vi "Main Screen_Hourly Cnt.vi"(9 "Current Date":string, 11 "connection reference 2":T1) -> (2 "Station Wise Max":i32[][](array[numeric]))   [LabVIEW 2017]
uses:
  <vilib>/addons/database/Connection.llb/Conn ObjectReference.ctl
  <vilib>/addons/database/Connection.llb/Conn Execute.vi
  <vilib>/addons/database/Recordset.llb/Rec Fetch Recordset Data (R).vi
  <vilib>/addons/database/Recordset.llb/Rec Destroy - Connection.vi
  <vilib>/addons/database/NI_Database_API.lvlib
panel:
  out "All Max":i32[](array[numeric])
  out "Table":string[][][](array[string])
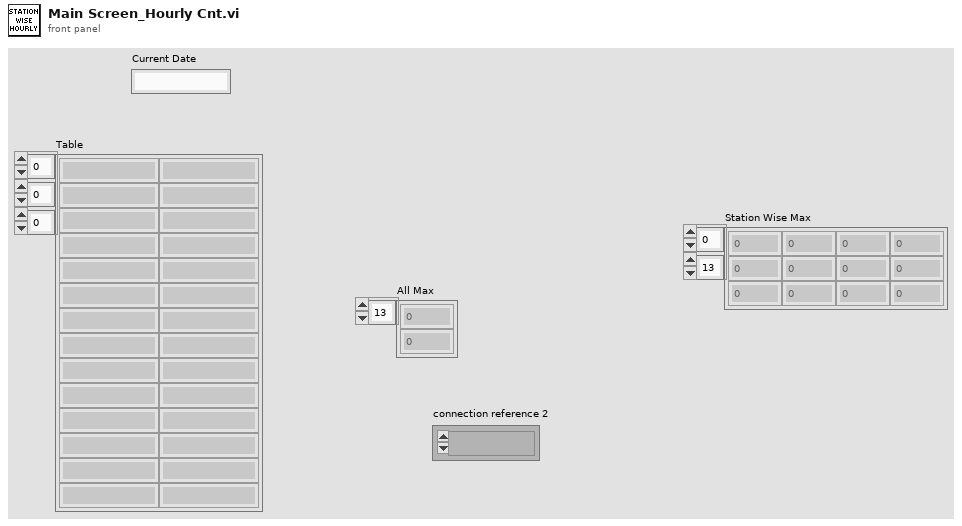
[diagram p1: front panel]
types:
  T1 = typedef "NI_Database_API.lvlib/Conn ObjectReference.ctl" = refnum<k1>
  T2 = typedef "NI_Database_API.lvlib/Rec ObjectReference.ctl" = refnum<k1>
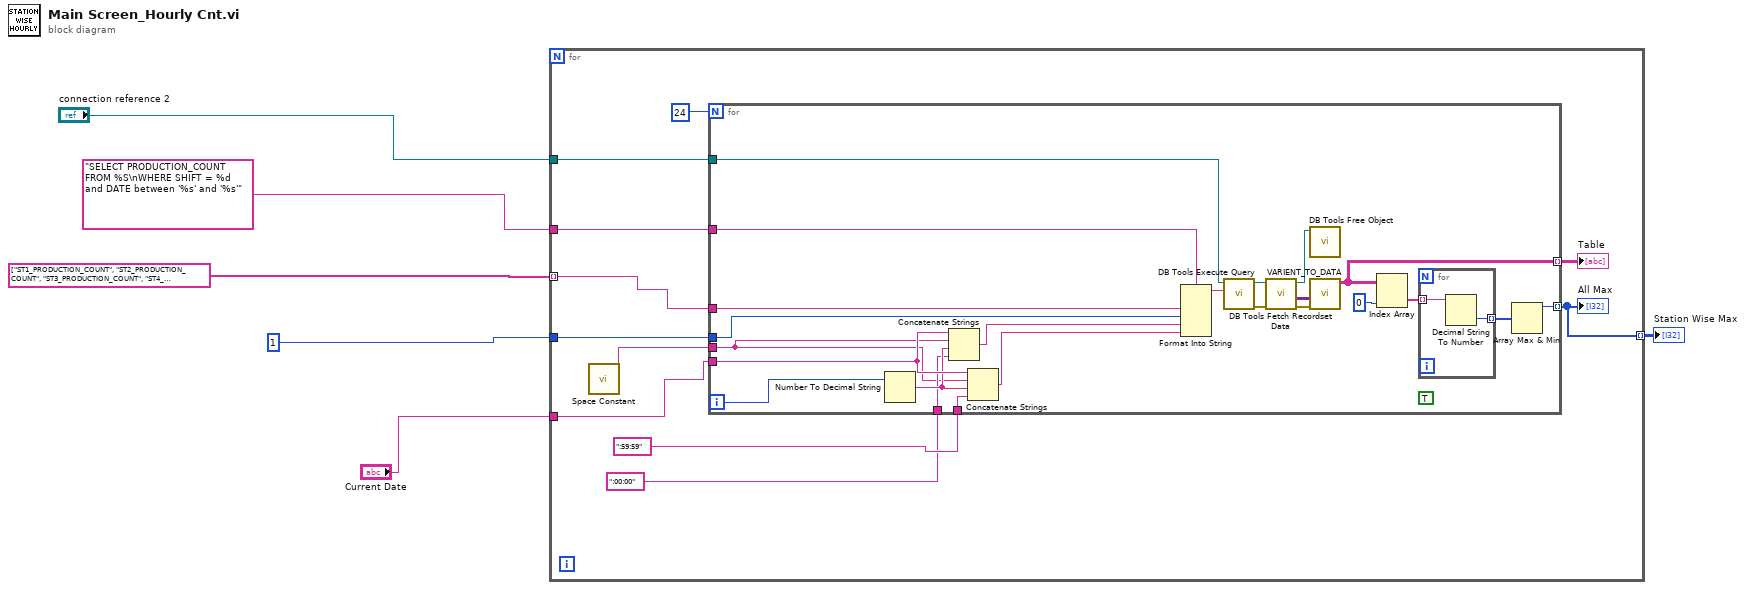
[diagram p0: block diagram]
diagram:
  n1 = for {
    tunnel: "SELECT PRODUCTION_COUNT FROM %S\nWHERE SHIFT = %d and DATE between '%s' and '%s'" ("SQL query") -> [w17]
    tunnel: 1 -> [w16]
    tunnel: "connection reference 2" -> [w15]
    tunnel: string[] ["ST1_PRODUCTION_COUNT", "ST2_PRODUCTION_COUNT", "ST3_PRODUCTION_COUNT", "ST4_PRODUCTION_COUNT", "ST5_PRODUCTION_COUNT", "ST6_PRODUCTION_COUNT"] -> [w10] mode=indexing
    tunnel: [w9] -> w2 mode=indexing
    tunnel: "Current Date" -> [w8]
    n2 = call <vilib>:"Space Constant.vi"() -> ("String"=w7:string)
    n3 = for {
      N: 24 -> [_]
      tunnel: w15 -> [w40]
      tunnel: w17 -> [w36]
      tunnel: w10 -> [w32]
      tunnel: w16 -> [w31]
      tunnel: w8 -> [w23]
      tunnel: [w29] -> w13 mode=indexing
      tunnel: [w30] -> w9 mode=indexing
      tunnel: ":59:59" -> [w24]
      tunnel: ":00:00" -> [w21]
      tunnel: w7 -> [w18]
      i -> [w19]
      (unwired) TRUE ("Check Hourly")
      n4 = Number To Decimal String(number=w19) -> (decimal integer string=w22:string)  [unwired: 1 in]
      n5 = Concatenate Strings(w23, w18, w22, w21) -> (w20:string)
      n6 = Concatenate Strings(w23, w18, w22, w24) -> (w25:string)
      n7 = Format Into String(format string=w36, w32, w31, w20, w25) -> (resulting string=w35:string)  [unwired: 2 in, 1 out]
      n8 = call-poly <vilib>:"DB Tools Execute Query.vi"("SQL query"=w35, "connection reference"=w40) -> ("error out"=w34:errorcluster, "recordset reference"=w39:T2)  [unwired: 6 in]
      n9 = call-poly <vilib>:"DB Tools Fetch Recordset Data.vi"("error in (no error)"=w34, "recordset reference"=w39) -> ("error out"=w33:errorcluster, "recordset data"=w37:variant[][], "recordset reference out"=w38:T2)  [unwired: 3 in]
      n10 = call-poly <vilib>:"DB Tools Free Object.vi"("recordset reference"=w38) -> ()  [unwired: 9 in, 2 out]
      n11 = call "VARIENT_TO_DATA.vi"("data"=w37, "error in (no error)"=w33) -> ("Table"=w29:string[][])  [unwired: 7 in, 1 out]
      n12 = Index Array(array=w29, index (col)=0 ("disabled index (col)")) -> (element=w27:string[])  [unwired: 1 in]
      n13 = for {
        tunnel: w27 -> [w42] mode=indexing
        tunnel: [w41] -> w26 mode=indexing
        n14 = Decimal String To Number(string=w42) -> (number=w41:i32)  [unwired: 2 in, 1 out]
      }
      n15 = Array Max & Min(array=w26) -> (max value=w30:i32)  [unwired: 3 out]
    }
    "Table" <- w13
    "All Max" <- w9
  }
  "Station Wise Max" <- w2
